vi "DB_Alarmas.vi"(8 "error in (no error)":errorcluster, 9 "Final":timestamp, 10 "Inicio":timestamp) -> (0 "error out":errorcluster, 3 "Data":string[][](array[string]))   [LabVIEW 2018]
uses:
  <vilib>/addons/database/Connection.llb/DB Tools Open Connec (Path).vi
  <vilib>/addons/database/Connection.llb/Conn Execute.vi
  <vilib>/addons/database/Recordset.llb/Rec Fetch Recordset Data (R).vi
  <vilib>/addons/database/Recordset.llb/Rec Destroy - Connection.vi
  <vilib>/addons/database/_DB Variant To Data/Database Variant To Data.xnode
  <vilib>/addons/database/NI_Database_API.lvlib
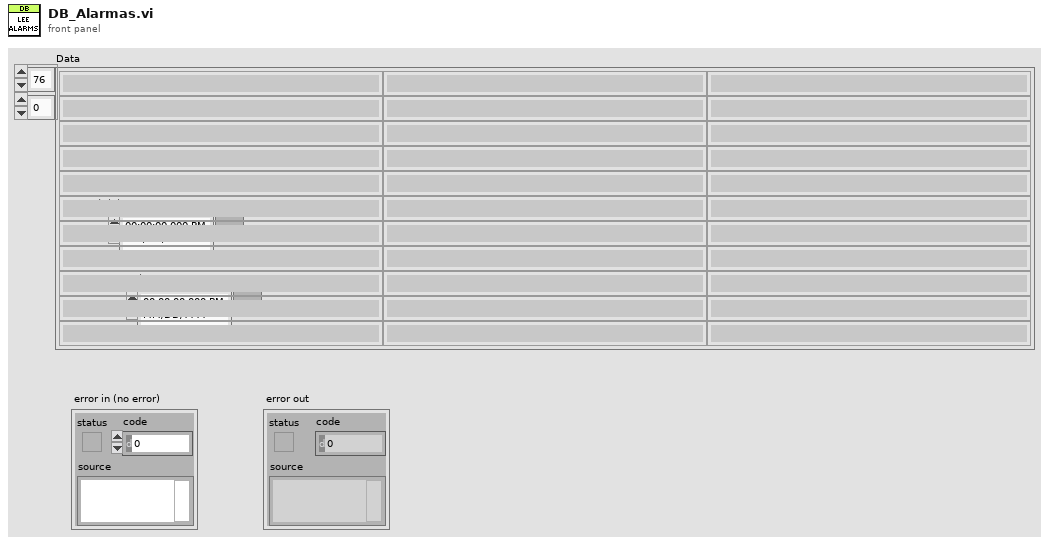
[diagram p1: front panel]
types:
  T1 = typedef "NI_Database_API.lvlib/Conn ObjectReference.ctl" = refnum<k1>
  T2 = typedef "NI_Database_API.lvlib/Rec ObjectReference.ctl" = refnum<k1>
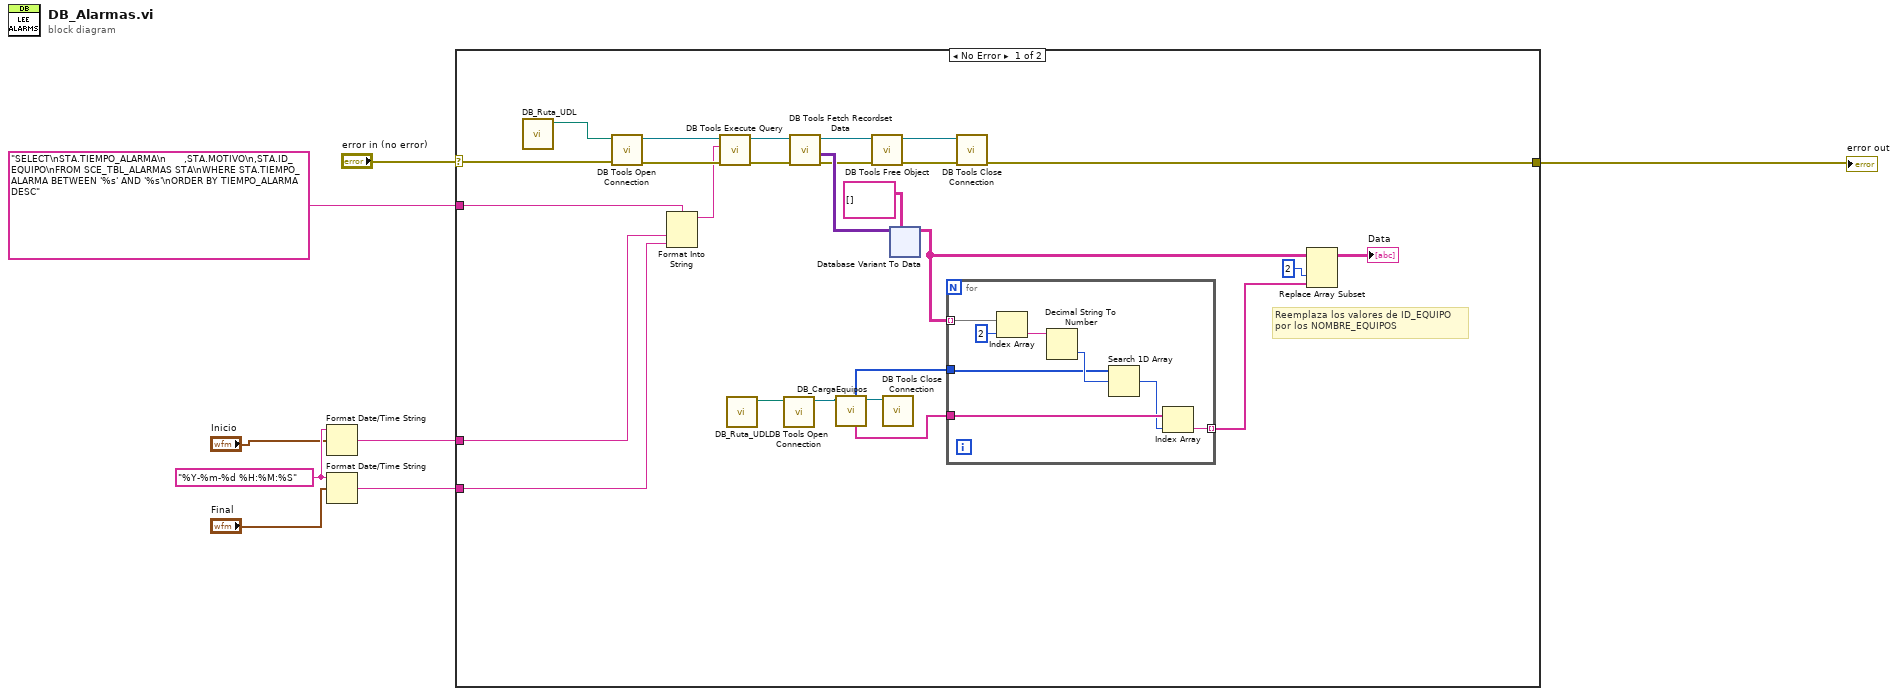
[diagram p0: block diagram]
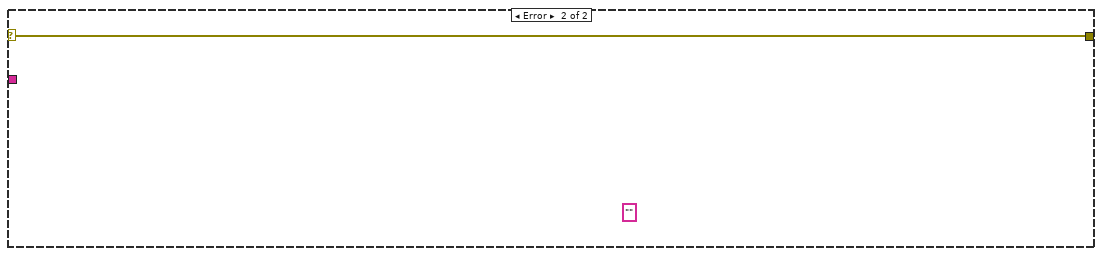
[diagram p2: hidden frame]
diagram:
  w6 = "%Y-%m-%d %H:%M:%S" ("time format string (%c)")
  n1 = Format Date/Time String(time format string (%c)=w6, seconds (now)="Inicio") -> (date/time string=w3:string)  [unwired: 1 in]
  n2 = Format Date/Time String(time format string (%c)=w6, seconds (now)="Final") -> (date/time string=w2:string)  [unwired: 1 in]
  n3 = case shown="No Error" "error in (no error)" {
    selector: "error in (no error)" -> [w29 w87]
    tunnel: [w31 w87] -> w7
    tunnel: "SELECT\nSTA.TIEMPO_ALARMA\n      ,STA.MOTIVO\n,STA.ID_EQUIPO\nFROM SCE_TBL_ALARMAS STA\nWHERE STA.TIEMPO_ALARMA BETWEEN '%s' AND '%s'\nORDER BY TIEMPO_ALARMA DESC" ("SQL") -> [w23 _]
    tunnel: w3 -> [w21 _]
    tunnel: w2 -> [w20 _]
    frame No Error {
      # "Reemplaza los valores de ID_EQUIPO\npor los NOMBRE_EQUIPOS"
      n4 = call "DB_Ruta_UDL.vi"() -> ("UDL ruta"=w19:path)  [unwired: 11 in]
      n5 = call-poly <vilib>:"DB Tools Open Connection.vi"("error in (no error)"=w29, "connection information"=w19) -> ("error out"=w34:errorcluster, "connection reference"=w32:T1)  [unwired: 6 in]
      n6 = Format Into String(format string=w23, w21, w20) -> (resulting string=w22:string)  [unwired: 2 in, 1 out]
      n7 = call-poly <vilib>:"DB Tools Execute Query.vi"("error in (no error)"=w34, "SQL query"=w22, "connection reference"=w32) -> ("error out"=w30:errorcluster, "recordset reference"=w28:T2)  [unwired: 5 in]
      n8 = call "DB_Ruta_UDL.vi"() -> ("UDL ruta"=w17:path)  [unwired: 11 in]
      n9 = call-poly <vilib>:"DB Tools Open Connection.vi"("connection information"=w17) -> ("connection reference"=w16:T1)  [unwired: 7 in, 1 out]
      n10 = call-poly <vilib>:"DB Tools Fetch Recordset Data.vi"("error in (no error)"=w30, "recordset reference"=w28) -> ("error out"=w24:errorcluster, "recordset data"=w25:variant[][], "recordset reference out"=w27:T2)  [unwired: 3 in]
      n11 = call "DB_CargaEquipos.vi"("db in"=w16) -> ("db out"=w15:T1, "NOMBRE_EQUIPOS"=w13:string[], "ID_EQUIPOS"=w14:i32[])  [unwired: 3 in, 5 out]
      n12 = call-poly <vilib>:"DB Tools Free Object.vi"("error in (no error)"=w24, "recordset reference"=w27) -> ("error out"=w33:errorcluster, "connection reference"=w18:T1)  [unwired: 8 in]
      n13 = call <vilib>:"DB Tools Close Connection.vi"("connection reference"=w15) -> ()  [unwired: 6 in, 1 out]
      n14 = xnode "Database Variant To Data"("database variant"=w25, "type"=string[][] []) -> ("data"=w12:string[][])  [unwired: 1 in, 1 out]
      n15 = for {
        tunnel: w12 -> [w42] mode=indexing
        tunnel: w14 -> [w38]
        tunnel: w13 -> [w37]
        tunnel: [w35] -> w10 mode=indexing
        n16 = Index Array(array=w42, index=2) -> (element=w40:string)
        n17 = Decimal String To Number(string=w40) -> (number=w39:i32)  [unwired: 2 in, 1 out]
        n18 = Search 1D Array(1D array=w38, element=w39) -> (index of element=w36:i32)  [unwired: 1 in]
        n19 = Index Array(array=w37, index=w36) -> (element=w35:string)
      }
      n20 = call <vilib>:"DB Tools Close Connection.vi"("error in (no error)"=w33, "connection reference"=w18) -> ("error out"=w31:errorcluster)  [unwired: 5 in]
      n21 = Replace Array Subset(array=w12, new element=w10, index (col)=2 ("disabled index (col)")) -> (→"Data":string[][])  [unwired: 1 in]
    }
    frame Error {
      (unwired) ""
    }
  }
  "error out" <- w7
